vi "Account Information.vi"(8 "error in (no error)":errorcluster, 10 "Password":string, 11 "file path (dialog if empty)":path) -> (0 "error out":errorcluster, 3 "Account Information":T1)   [LabVIEW 2020]
doc: "This VI extract the account information: Name, balance and password."
uses:
  <vilib>/Utility/file.llb/Read Delimited Spreadsheet (string).vi
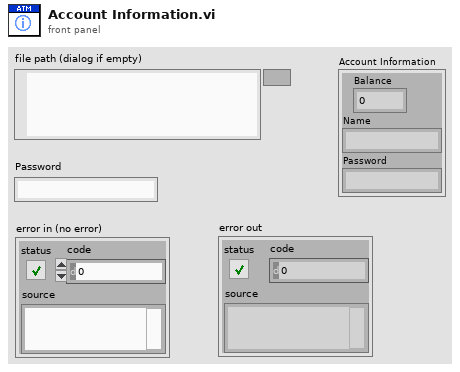
[diagram p1: front panel]
types:
  T1 = cluster{"Balance":dbl, "Name":string, "Password":string}
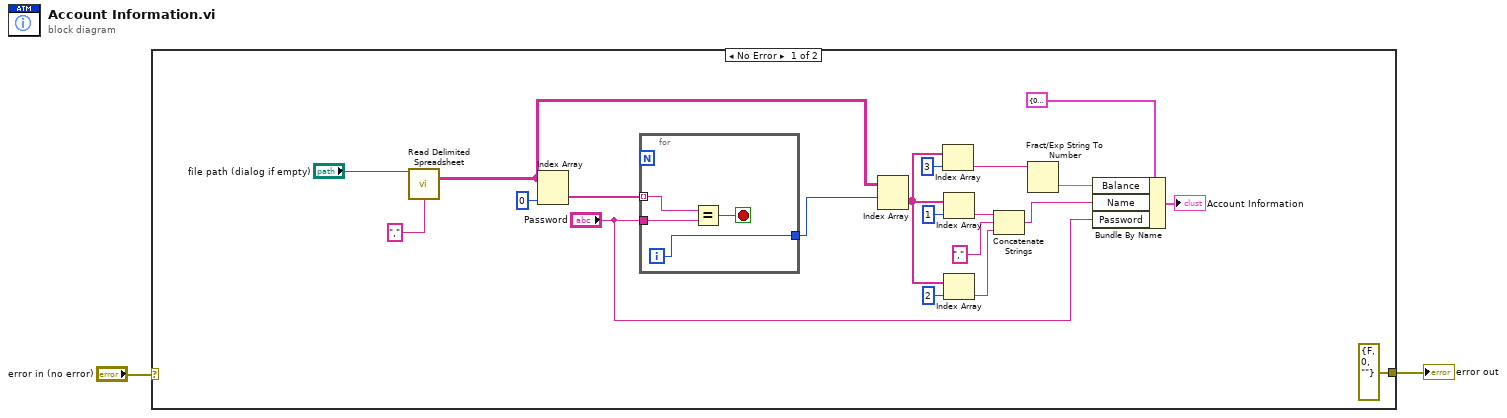
[diagram p0: block diagram]
diagram:
  n1 = case shown="No Error" "error in (no error)" {
    selector: "error in (no error)" -> [_ w27]
    tunnel: [errorcluster {"status"=FALSE, "code"=0, "source"=""} ("error IO") w27] -> w2
    frame No Error {
      n2 = call-poly <vilib>:"Read Delimited Spreadsheet.vi"("file path (dialog if empty)"="file path (dialog if empty)", "delimiter (\\t)"="," ("delimiter (\\t)")) -> ("all rows"=w18:string[][])  [unwired: 8 in, 5 out]
      n3 = Index Array(array=w18, index (col)=0 ("disabled index (col)")) -> (element=w19:string[])  [unwired: 1 in]
      n4 = for {
        tunnel: "Password" -> [w26]
        tunnel: w19 -> [w24] mode=indexing
        tunnel: [w23] -> w17
        i -> [w23]
        stop <- w25 stop-if-true
        n5 = Equal?(x=w24, y=w26) -> (x = y?=w25:bool)
      }
      n6 = Index Array(array=w18, index (row)=w17) -> (element=w9:string[])  [unwired: 1 in]
      n7 = Index Array(array=w9, index=3) -> (element=w7:string)
      n8 = Index Array(array=w9, index=1) -> (element=w14:string)
      n9 = Index Array(array=w9, index=2) -> (element=w11:string)
      n10 = Concatenate Strings(w14, "," ("string"), w11) -> (w10:string)
      n11 = Fract/Exp String To Number(string=w7) -> (number=w6:dbl)  [unwired: 3 in, 1 out]
      n12 = Bundle By Name(cluster=T1 {"Balance"=0.0, "Name"="", "Password"=""}, "Balance"=w6, "Name"=w10, "Password"="Password") -> (→"Account Information":T1)
    }
    frame Error {
    }
  }
  "error out" <- w2
